vi "real time object finder single cam with save v1.0 EJA 09 14 2016.vi"() -> ()   [LabVIEW 2015]
doc: "The Low-Level Grab VI acquires images continuously and displays the images in an image control using low-level acquisition VIs. A grab is appropriate for high-speed applications in which you need to process only one image at a time."
uses:
  <vilib>/userdefined/High Color/IMAQdx.ctl
  <vilib>/vision/driver/IMAQdx.llb/IMAQdx Buffer Number Mode.ctl
  <vilib>/Utility/file.llb/Write To Spreadsheet File (DBL).vi
  <vilib>/vision/driver/NI_Vision_Acquisition_Software.lvlib
  <resource>/objmgr/imaqdx.rc
  <vilib>/Analysis/NI_AALBase.lvlib
panel:
  out "y position histogram":T1(graph)={"X Values"=[496.25, 512.75, 529.25, 545.75, 562.25, 578.75, 595.25, 611.75, 628.25, 644.75], "Histogram: h(x)"=[12, 8, 7, 11, 11, 133, 43, 197, 42, 41]}
  out "x position histogram":T1(graph)={"X Values"=[593.75, 617.25, 640.75, 664.25, 687.75, 711.25, 734.75, 758.25, 781.75, 805.25], "Histogram: h(x)"=[96, 9, 49, 4, 6, 45, 112, 75, 70, 39]}
  in  "histogram \nbins":i32=10
  in  "always save\non stop\nimaging":bool=TRUE
  in  "acquisition \ntime (s)":i32=5
  in  "save for a \ndesignated \nperiod":bool
  out "trajectory":cluster{i32[], i32[]}(graph)={[740, 740, 740, 740, 740, 740, 740, 740, 740, 740, 740, 740, 740, 740, 740, 740, 740, 740, 740, 740, 740, 740, 740, 740, 740, 740, 740, 740, 740, 740, 740, 740, 740, 740, 740, 740, 740, 740, 740, 740, 740, 740, 740, 740, 740, 740, 740, 740, 740, 741, 742, 744, 747, 749, 751, 752, 753, 755, 757, 759, 760, 763, 766, 771, 776, 779, 783, 787, 789, 790, 791, 791, 791, 790, 788, 785, 782, 778, 775, 773, 771, 770, 769, 767, 765, 763, 760, 755, 749, 744, 740, 736, 733, 730, 727, 725, 724, 723, 722, 722, 723, 726, 730, 733, 738, 743, 748, 752, 756, 758, 761, 764, 768, 770, 772, 776, 780, 783, 786, 788, 790, 790, 790, 789, 788, 786, 784, 781, 779, 776, 773, 769, 765, 760, 753, 746, 740, 735, 730, 725, 723, 721, 717, 713, 710, 707, 705, 703, 701, 700, 701, 701, 703, 705, 707, 710, 713, 718, 723, 728, 733, 738, 743, 750, 758, 762, 763, 765, 767, 769, 771, 773, 773, 773, 771, 769, 766, 763, 759, 756, 752, 749, 746, 743, 739, 736, 732, 727, 725, 724, 721, 719, 716, 714, 713, 712, 711, 710, 709, 709, 710, 710, 712, 715, 718, 721, 724, 728, 733, 740, 748, 755, 759, 763, 769, 773, 776, 779, 780, 780, 781, 780, 779, 778, 777, 775, 774, 772, 769, 769, 768, 766, 764, 762, 758, 755, 753, 748, 744, 741, 739, 734, 730, 727, 725, 723, 722, 722, 722, 722, 723, 724, 727, 729, 731, 734, 737, 741, 746, 750, 754, 757, 762, 764, 765, 765, 765, 765, 765, 767, 771, 776, 777, 780, 783, 785, 787, 790, 792, 794, 797, 798, 801, 804, 806, 808, 810, 811, 812, 814, 816, 817, 817, 817, 817, 817, 817, 817, 817, 817, 817, 817, 817, 817, 817, 817, 817, 817, 817, 817, 817, 817, 815, 813, 808, 804, 799, 794, 791, 789, 785, 782, 777, 772, 768, 765, 762, 759, 754, 747, 743, 739, 734, 728, 723, 719, 715, 711, 708, 705, 701, 697, 693, 689, 684, 681, 677, 673, 667, 658, 654, 652, 650, 647, 642, 640, 640, 638, 637, 637, 637, 637, 637, 637, 637, 636, 636, 636, 635, 635, 635, 635, 635, 634, 634, 633, 633, 633, 633, 633, 633, 633, 633, 634, 634, 635, 635, 636, 636, 637, 637, 638, 638, 639, 639, 639, 638, 634, 631, 629, 626, 623, 619, 616, 614, 612, 610, 608, 607, 605, 602, 600, 599, 597, 594, 592, 591, 589, 588, 587, 586, 585, 584, 583, 582, 582, 582, 582, 582, 582, 582, 584, 585, 585, 585, 585, 585, 585, 585, 585, 585, 585, 585, 585, 585, 585, 585, 585, 585, 585, 585, 585, 585, 585, 585, 585, 585, 585, 585, 585, 585, 585, 585, 585, 585, 585, 585, 585, 585, 585, 585, 585, 585, 585, 585, 585, 585, 585, 585, 585, 585, 585, 585, 585, 585, 585, 585, 585, 585, 585, 585, 585, 585, 585, 585, 585, 585, 585, 585, 585, 585, 585, 585, 585, 585], [615, 618, 617, 617, 617, 618, 617, 617, 617, 618, 618, 617, 617, 618, 618, 617, 618, 617, 618, 617, 619, 617, 618, 615, 617, 618, 618, 617, 619, 618, 618, 618, 618, 619, 617, 615, 617, 617, 615, 617, 618, 617, 617, 615, 615, 617, 617, 619, 618, 615, 614, 613, 613, 610, 610, 609, 608, 607, 607, 609, 608, 612, 612, 615, 616, 620, 622, 625, 620, 628, 630, 631, 633, 636, 639, 643, 647, 651, 652, 653, 653, 653, 653, 652, 653, 653, 652, 651, 647, 646, 644, 642, 644, 637, 636, 633, 633, 630, 625, 625, 622, 619, 616, 611, 607, 605, 604, 603, 602, 604, 602, 603, 601, 602, 604, 607, 610, 613, 616, 619, 622, 625, 628, 631, 636, 638, 639, 638, 639, 639, 642, 643, 643, 643, 645, 643, 644, 644, 646, 645, 650, 643, 646, 644, 640, 639, 636, 631, 627, 625, 620, 617, 614, 610, 607, 599, 596, 593, 591, 589, 584, 583, 584, 584, 583, 585, 588, 587, 589, 593, 598, 601, 602, 607, 610, 616, 618, 620, 622, 623, 625, 624, 629, 624, 624, 628, 625, 627, 625, 625, 624, 622, 625, 616, 614, 616, 613, 611, 607, 604, 595, 592, 590, 588, 586, 584, 583, 579, 576, 575, 576, 577, 579, 577, 580, 583, 585, 590, 592, 596, 599, 602, 608, 608, 612, 611, 612, 615, 615, 615, 616, 616, 616, 614, 616, 615, 617, 615, 613, 609, 609, 607, 604, 602, 600, 597, 595, 593, 591, 590, 589, 585, 587, 584, 583, 584, 579, 578, 576, 575, 574, 576, 572, 572, 575, 573, 575, 575, 573, 573, 574, 578, 576, 577, 578, 578, 581, 581, 581, 582, 583, 583, 584, 585, 579, 586, 587, 586, 583, 583, 583, 583, 583, 583, 583, 583, 583, 583, 583, 583, 583, 583, 583, 583, 583, 583, 583, 583, 583, 583, 583, 587, 583, 582, 586, 585, 585, 584, 584, 583, 583, 583, 582, 581, 583, 583, 580, 581, 581, 581, 579, 579, 578, 577, 576, 576, 580, 579, 579, 576, 577, 577, 577, 576, 576, 580, 575, 574, 578, 577, 575, 575, 575, 575, 576, 575, 575, 576, 575, 575, 575, 575, 574, 573, 570, 568, 564, 562, 560, 558, 555, 553, 549, 547, 545, 543, 541, 540, 538, 535, 530, 525, 525, 517, 517, 515, 507, 509, 503, 497, 499, 492, 490, 488, 488, 488, 489, 495, 498, 503, 509, 514, 519, 525, 530, 535, 541, 545, 550, 554, 558, 562, 567, 571, 576, 580, 583, 587, 593, 595, 598, 602, 605, 608, 611, 612, 612, 612, 612, 611, 612, 610, 609, 609, 609, 609, 609, 609, 609, 609, 609, 609, 609, 609, 609, 609, 609, 609, 609, 608, 609, 609, 609, 610, 609, 609, 609, 609, 609, 609, 609, 610, 609, 610, 609, 609, 613, 609, 613, 609, 609, 609, 611, 609, 609, 609, 609, 609, 608, 609, 609, 609, 609, 609, 609, 609, 609, 609, 609, 609, 609, 609, 609, 609, 609, 609, 609, 609, 609, 611, 609, 609, 609, 609, 608]}
  in  "save\nlast\nimage":bool
  in  "stop no save":bool
  out "date stub assigned":string="_2018Y_03M_05D_11h_28m_40s"
  in  "Acquire\ndata":bool
  in  "Experimental stub":string="test01_test"
  out "Saving":bool
  in  "save data":bool
  in  "save path":path=path "C:/Users/StangebyeTO1/OneDrive/Documents/RasterImageLabview/object_tracker"
  in  "number\nformat (%.6f)":string="%.6f"
  in  "Marker\nText color":u32(colorbox)=16711680
  out "Multiplot":cluster{cluster{dbl, i32}[]}[](graph)=[{[{0.0, 740}, {0.025, 740}, {0.049, 740}, {0.073, 740}, {0.097, 740}, {0.122, 740}, {0.145, 740}, {0.171, 740}, {0.194, 740}, {0.218, 740}, {0.242, 740}, {0.266, 740}, {0.29, 740}, {0.313, 740}, {0.338, 740}, {0.361, 740}, {0.385, 740}, {0.41, 740}, {0.434, 740}, {0.458, 740}, {0.483, 740}, {0.506, 740}, {0.53, 740}, {0.556, 740}, {0.578, 740}, {0.602, 740}, {0.626, 740}, {0.651, 740}, {0.674, 740}, {0.698, 740}, {0.722, 740}, {0.746, 740}, {0.771, 740}, {0.794, 740}, {0.819, 740}, {0.842, 740}, {0.867, 740}, {0.89, 740}, {0.915, 740}, {0.939, 740}, {0.963, 740}, {0.987, 740}, {1.011, 740}, {1.035, 740}, {1.059, 740}, {1.083, 740}, {1.107, 740}, {1.132, 740}, {1.157, 740}, {1.179, 741}, {1.204, 742}, {1.227, 744}, {1.251, 747}, {1.275, 749}, {1.3, 751}, {1.323, 752}, {1.348, 753}, {1.372, 755}, {1.396, 757}, {1.42, 759}, {1.444, 760}, {1.468, 763}, {1.492, 766}, {1.516, 771}, {1.54, 776}, {1.564, 779}, {1.588, 783}, {1.612, 787}, {1.637, 789}, {1.66, 790}, {1.685, 791}, {1.708, 791}, {1.733, 791}, {1.756, 790}, {1.78, 788}, {1.805, 785}, {1.828, 782}, {1.853, 778}, {1.876, 775}, {1.901, 773}, {1.925, 771}, {1.95, 770}, {1.973, 769}, {1.997, 767}, {2.021, 765}, {2.045, 763}, {2.07, 760}, {2.093, 755}, {2.118, 749}, {2.141, 744}, {2.166, 740}, {2.189, 736}, {2.213, 733}, {2.237, 730}, {2.261, 727}, {2.286, 725}, {2.31, 724}, {2.334, 723}, {2.357, 722}, {2.382, 722}, {2.406, 723}, {2.429, 726}, {2.454, 730}, {2.478, 733}, {2.503, 738}, {2.526, 743}, {2.55, 748}, {2.574, 752}, {2.598, 756}, {2.622, 758}, {2.646, 761}, {2.671, 764}, {2.694, 768}, {2.718, 770}, {2.743, 772}, {2.767, 776}, {2.791, 780}, {2.814, 783}, {2.838, 786}, {2.863, 788}, {2.886, 790}, {2.91, 790}, {2.935, 790}, {2.959, 789}, {2.984, 788}, {3.007, 786}, {3.031, 784}, {3.055, 781}, {3.079, 779}, {3.104, 776}, {3.127, 773}, {3.152, 769}, {3.175, 765}, {3.2, 760}, {3.225, 753}, {3.249, 746}, {3.272, 740}, {3.295, 735}, {3.32, 730}, {3.343, 725}, {3.368, 723}, {3.391, 721}, {3.415, 717}, {3.44, 713}, {3.463, 710}, {3.487, 707}, {3.512, 705}, {3.536, 703}, {3.56, 701}, {3.584, 700}, {3.608, 701}, {3.632, 701}, {3.657, 703}, {3.68, 705}, {3.704, 707}, {3.728, 710}, {3.753, 713}, {3.776, 718}, {3.801, 723}, {3.824, 728}, {3.849, 733}, {3.872, 738}, {3.897, 743}, {3.921, 750}, {3.944, 758}, {3.969, 762}, {3.993, 763}, {4.017, 765}, {4.04, 767}, {4.064, 769}, {4.089, 771}, {4.113, 773}, {4.138, 773}, {4.162, 773}, {4.186, 771}, {4.209, 769}, {4.234, 766}, {4.257, 763}, {4.281, 759}, {4.306, 756}, {4.33, 752}, {4.354, 749}, {4.377, 746}, {4.401, 743}, {4.426, 739}, {4.45, 736}, {4.474, 732}, {4.498, 727}, {4.522, 725}, {4.546, 724}, {4.57, 721}, {4.594, 719}, {4.618, 716}, {4.641, 714}, {4.668, 713}, {4.69, 712}, {4.714, 711}, {4.738, 710}, {4.762, 709}, {4.787, 709}, {4.81, 710}, {4.834, 710}, {4.86, 712}, {4.883, 715}, {4.906, 718}, {4.93, 721}, {4.955, 724}, {4.979, 728}, {5.003, 733}, {5.027, 740}, {5.051, 748}, {5.075, 755}, {5.099, 759}, {5.123, 763}, {5.147, 769}, {5.172, 773}, {5.195, 776}, {5.22, 779}, {5.245, 780}, {5.268, 780}, {5.291, 781}, {5.315, 780}, {5.339, 779}, {5.363, 778}, {5.388, 777}, {5.411, 775}, {5.436, 774}, {5.46, 772}, {5.484, 769}, {5.508, 769}, {5.531, 768}, {5.555, 766}, {5.58, 764}, {5.604, 762}, {5.628, 758}, {5.652, 755}, {5.676, 753}, {5.7, 748}, {5.724, 744}, {5.748, 741}, {5.772, 739}, {5.796, 734}, {5.821, 730}, {5.844, 727}, {5.868, 725}, {5.892, 723}, {5.917, 722}, {5.94, 722}, {5.966, 722}, {5.989, 722}, {6.013, 723}, {6.037, 724}, {6.06, 727}, {6.085, 729}, {6.108, 731}, {6.133, 734}, {6.158, 737}, {6.181, 741}, {6.205, 746}, {6.229, 750}, {6.254, 754}, {6.277, 757}, {6.301, 762}, {6.325, 764}, {6.35, 765}, {6.373, 765}, {6.397, 765}, {6.423, 765}, {6.446, 765}, {6.471, 767}, {6.494, 771}, {6.518, 776}, {6.542, 777}, {6.567, 780}, {6.59, 783}, {6.614, 785}, {6.638, 787}, {6.662, 790}, {6.687, 792}, {6.71, 794}, {6.734, 797}, {6.758, 798}, {6.783, 801}, {6.806, 804}, {6.83, 806}, {6.854, 808}, {6.878, 810}, {6.903, 811}, {6.926, 812}, {6.951, 814}, {6.974, 816}, {6.999, 817}, {7.023, 817}, {7.048, 817}, {7.071, 817}, {7.094, 817}, {7.12, 817}, {7.143, 817}, {7.168, 817}, {7.191, 817}, {7.215, 817}, {7.239, 817}, {7.263, 817}, {7.287, 817}, {7.311, 817}, {7.336, 817}, {7.359, 817}, {7.384, 817}, {7.407, 817}, {7.432, 817}, {7.456, 817}, {7.479, 817}, {7.504, 815}, {7.528, 813}, {7.552, 808}, {7.576, 804}, {7.6, 799}, {7.624, 794}, {7.648, 791}, {7.672, 789}, {7.696, 785}, {7.721, 782}, {7.744, 777}, {7.769, 772}, {7.792, 768}, {7.817, 765}, {7.84, 762}, {7.864, 759}, {7.888, 754}, {7.912, 747}, {7.936, 743}, {7.96, 739}, {7.984, 734}, {8.009, 728}, {8.033, 723}, {8.056, 719}, {8.081, 715}, {8.105, 711}, {8.128, 708}, {8.153, 705}, {8.176, 701}, {8.201, 697}, {8.224, 693}, {8.249, 689}, {8.273, 684}, {8.297, 681}, {8.321, 677}, {8.345, 673}, {8.369, 667}, {8.393, 658}, {8.417, 654}, {8.441, 652}, {8.465, 650}, {8.489, 647}, {8.513, 642}, {8.537, 640}, {8.561, 640}, {8.585, 638}, {8.609, 637}, {8.634, 637}, {8.657, 637}, {8.681, 637}, {8.706, 637}, {8.73, 637}, {8.754, 637}, {8.778, 636}, {8.802, 636}, {8.826, 636}, {8.851, 635}, {8.874, 635}, {8.899, 635}, {8.922, 635}, {8.947, 635}, {8.971, 634}, {8.995, 634}, {9.02, 633}, {9.042, 633}, {9.066, 633}, {9.09, 633}, {9.114, 633}, {9.139, 633}, {9.162, 633}, {9.188, 633}, {9.211, 634}, {9.236, 634}, {9.259, 635}, {9.283, 635}, {9.307, 636}, {9.332, 636}, {9.355, 637}, {9.379, 637}, {9.404, 638}, {9.427, 638}, {9.451, 639}, {9.475, 639}, {9.5, 639}, {9.523, 638}, {9.547, 634}, {9.572, 631}, {9.595, 629}, {9.62, 626}, {9.643, 623}, {9.668, 619}, {9.691, 616}, {9.715, 614}, {9.739, 612}, {9.764, 610}, {9.788, 608}, {9.812, 607}, {9.837, 605}, {9.86, 602}, {9.884, 600}, {9.908, 599}, {9.932, 597}, {9.955, 594}, {9.98, 592}, {10.004, 591}, {10.028, 589}, {10.053, 588}, {10.076, 587}, {10.101, 586}, {10.124, 585}, {10.149, 584}, {10.172, 583}, {10.196, 582}, {10.221, 582}, {10.244, 582}, {10.269, 582}, {10.293, 582}, {10.317, 582}, {10.341, 582}, {10.365, 584}, {10.39, 585}, {10.412, 585}, {10.437, 585}, {10.461, 585}, {10.485, 585}, {10.509, 585}, {10.534, 585}, {10.557, 585}, {10.581, 585}, {10.605, 585}, {10.629, 585}, {10.654, 585}, {10.677, 585}, {10.701, 585}, {10.725, 585}, {10.75, 585}, {10.773, 585}, {10.797, 585}, {10.822, 585}, {10.845, 585}, {10.87, 585}, {10.893, 585}, {10.918, 585}, {10.942, 585}, {10.966, 585}, {10.99, 585}, {11.014, 585}, {11.038, 585}, {11.062, 585}, {11.088, 585}, {11.11, 585}, {11.135, 585}, {11.159, 585}, {11.182, 585}, {11.207, 585}, {11.231, 585}, {11.255, 585}, {11.279, 585}, {11.303, 585}, {11.326, 585}, {11.353, 585}, {11.375, 585}, {11.4, 585}, {11.423, 585}, {11.448, 585}, {11.471, 585}, {11.495, 585}, {11.52, 585}, {11.543, 585}, {11.569, 585}, {11.602, 585}, {11.621, 585}, {11.641, 585}, {11.664, 585}, {11.688, 585}, {11.711, 585}, {11.736, 585}, {11.76, 585}, {11.784, 585}, {11.808, 585}, {11.831, 585}, {11.856, 585}, {11.879, 585}, {11.904, 585}, {11.928, 585}, {11.952, 585}, {11.975, 585}, {12.0, 585}, {12.024, 585}, {12.047, 585}, {12.072, 585}, {12.096, 585}, {12.121, 585}]}, {[{0.0, 615}, {0.025, 618}, {0.049, 617}, {0.073, 617}, {0.097, 617}, {0.122, 618}, {0.145, 617}, {0.171, 617}, {0.194, 617}, {0.218, 618}, {0.242, 618}, {0.266, 617}, {0.29, 617}, {0.313, 618}, {0.338, 618}, {0.361, 617}, {0.385, 618}, {0.41, 617}, {0.434, 618}, {0.458, 617}, {0.483, 619}, {0.506, 617}, {0.53, 618}, {0.556, 615}, {0.578, 617}, {0.602, 618}, {0.626, 618}, {0.651, 617}, {0.674, 619}, {0.698, 618}, {0.722, 618}, {0.746, 618}, {0.771, 618}, {0.794, 619}, {0.819, 617}, {0.842, 615}, {0.867, 617}, {0.89, 617}, {0.915, 615}, {0.939, 617}, {0.963, 618}, {0.987, 617}, {1.011, 617}, {1.035, 615}, {1.059, 615}, {1.083, 617}, {1.107, 617}, {1.132, 619}, {1.157, 618}, {1.179, 615}, {1.204, 614}, {1.227, 613}, {1.251, 613}, {1.275, 610}, {1.3, 610}, {1.323, 609}, {1.348, 608}, {1.372, 607}, {1.396, 607}, {1.42, 609}, {1.444, 608}, {1.468, 612}, {1.492, 612}, {1.516, 615}, {1.54, 616}, {1.564, 620}, {1.588, 622}, {1.612, 625}, {1.637, 620}, {1.66, 628}, {1.685, 630}, {1.708, 631}, {1.733, 633}, {1.756, 636}, {1.78, 639}, {1.805, 643}, {1.828, 647}, {1.853, 651}, {1.876, 652}, {1.901, 653}, {1.925, 653}, {1.95, 653}, {1.973, 653}, {1.997, 652}, {2.021, 653}, {2.045, 653}, {2.07, 652}, {2.093, 651}, {2.118, 647}, {2.141, 646}, {2.166, 644}, {2.189, 642}, {2.213, 644}, {2.237, 637}, {2.261, 636}, {2.286, 633}, {2.31, 633}, {2.334, 630}, {2.357, 625}, {2.382, 625}, {2.406, 622}, {2.429, 619}, {2.454, 616}, {2.478, 611}, {2.503, 607}, {2.526, 605}, {2.55, 604}, {2.574, 603}, {2.598, 602}, {2.622, 604}, {2.646, 602}, {2.671, 603}, {2.694, 601}, {2.718, 602}, {2.743, 604}, {2.767, 607}, {2.791, 610}, {2.814, 613}, {2.838, 616}, {2.863, 619}, {2.886, 622}, {2.91, 625}, {2.935, 628}, {2.959, 631}, {2.984, 636}, {3.007, 638}, {3.031, 639}, {3.055, 638}, {3.079, 639}, {3.104, 639}, {3.127, 642}, {3.152, 643}, {3.175, 643}, {3.2, 643}, {3.225, 645}, {3.249, 643}, {3.272, 644}, {3.295, 644}, {3.32, 646}, {3.343, 645}, {3.368, 650}, {3.391, 643}, {3.415, 646}, {3.44, 644}, {3.463, 640}, {3.487, 639}, {3.512, 636}, {3.536, 631}, {3.56, 627}, {3.584, 625}, {3.608, 620}, {3.632, 617}, {3.657, 614}, {3.68, 610}, {3.704, 607}, {3.728, 599}, {3.753, 596}, {3.776, 593}, {3.801, 591}, {3.824, 589}, {3.849, 584}, {3.872, 583}, {3.897, 584}, {3.921, 584}, {3.944, 583}, {3.969, 585}, {3.993, 588}, {4.017, 587}, {4.04, 589}, {4.064, 593}, {4.089, 598}, {4.113, 601}, {4.138, 602}, {4.162, 607}, {4.186, 610}, {4.209, 616}, {4.234, 618}, {4.257, 620}, {4.281, 622}, {4.306, 623}, {4.33, 625}, {4.354, 624}, {4.377, 629}, {4.401, 624}, {4.426, 624}, {4.45, 628}, {4.474, 625}, {4.498, 627}, {4.522, 625}, {4.546, 625}, {4.57, 624}, {4.594, 622}, {4.618, 625}, {4.641, 616}, {4.668, 614}, {4.69, 616}, {4.714, 613}, {4.738, 611}, {4.762, 607}, {4.787, 604}, {4.81, 595}, {4.834, 592}, {4.86, 590}, {4.883, 588}, {4.906, 586}, {4.93, 584}, {4.955, 583}, {4.979, 579}, {5.003, 576}, {5.027, 575}, {5.051, 576}, {5.075, 577}, {5.099, 579}, {5.123, 577}, {5.147, 580}, {5.172, 583}, {5.195, 585}, {5.22, 590}, {5.245, 592}, {5.268, 596}, {5.291, 599}, {5.315, 602}, {5.339, 608}, {5.363, 608}, {5.388, 612}, {5.411, 611}, {5.436, 612}, {5.46, 615}, {5.484, 615}, {5.508, 615}, {5.531, 616}, {5.555, 616}, {5.58, 616}, {5.604, 614}, {5.628, 616}, {5.652, 615}, {5.676, 617}, {5.7, 615}, {5.724, 613}, {5.748, 609}, {5.772, 609}, {5.796, 607}, {5.821, 604}, {5.844, 602}, {5.868, 600}, {5.892, 597}, {5.917, 595}, {5.94, 593}, {5.966, 591}, {5.989, 590}, {6.013, 589}, {6.037, 585}, {6.06, 587}, {6.085, 584}, {6.108, 583}, {6.133, 584}, {6.158, 579}, {6.181, 578}, {6.205, 576}, {6.229, 575}, {6.254, 574}, {6.277, 576}, {6.301, 572}, {6.325, 572}, {6.35, 575}, {6.373, 573}, {6.397, 575}, {6.423, 575}, {6.446, 573}, {6.471, 573}, {6.494, 574}, {6.518, 578}, {6.542, 576}, {6.567, 577}, {6.59, 578}, {6.614, 578}, {6.638, 581}, {6.662, 581}, {6.687, 581}, {6.71, 582}, {6.734, 583}, {6.758, 583}, {6.783, 584}, {6.806, 585}, {6.83, 579}, {6.854, 586}, {6.878, 587}, {6.903, 586}, {6.926, 583}, {6.951, 583}, {6.974, 583}, {6.999, 583}, {7.023, 583}, {7.048, 583}, {7.071, 583}, {7.094, 583}, {7.12, 583}, {7.143, 583}, {7.168, 583}, {7.191, 583}, {7.215, 583}, {7.239, 583}, {7.263, 583}, {7.287, 583}, {7.311, 583}, {7.336, 583}, {7.359, 583}, {7.384, 583}, {7.407, 583}, {7.432, 583}, {7.456, 583}, {7.479, 587}, {7.504, 583}, {7.528, 582}, {7.552, 586}, {7.576, 585}, {7.6, 585}, {7.624, 584}, {7.648, 584}, {7.672, 583}, {7.696, 583}, {7.721, 583}, {7.744, 582}, {7.769, 581}, {7.792, 583}, {7.817, 583}, {7.84, 580}, {7.864, 581}, {7.888, 581}, {7.912, 581}, {7.936, 579}, {7.96, 579}, {7.984, 578}, {8.009, 577}, {8.033, 576}, {8.056, 576}, {8.081, 580}, {8.105, 579}, {8.128, 579}, {8.153, 576}, {8.176, 577}, {8.201, 577}, {8.224, 577}, {8.249, 576}, {8.273, 576}, {8.297, 580}, {8.321, 575}, {8.345, 574}, {8.369, 578}, {8.393, 577}, {8.417, 575}, {8.441, 575}, {8.465, 575}, {8.489, 575}, {8.513, 576}, {8.537, 575}, {8.561, 575}, {8.585, 576}, {8.609, 575}, {8.634, 575}, {8.657, 575}, {8.681, 575}, {8.706, 574}, {8.73, 573}, {8.754, 570}, {8.778, 568}, {8.802, 564}, {8.826, 562}, {8.851, 560}, {8.874, 558}, {8.899, 555}, {8.922, 553}, {8.947, 549}, {8.971, 547}, {8.995, 545}, {9.02, 543}, {9.042, 541}, {9.066, 540}, {9.09, 538}, {9.114, 535}, {9.139, 530}, {9.162, 525}, {9.188, 525}, {9.211, 517}, {9.236, 517}, {9.259, 515}, {9.283, 507}, {9.307, 509}, {9.332, 503}, {9.355, 497}, {9.379, 499}, {9.404, 492}, {9.427, 490}, {9.451, 488}, {9.475, 488}, {9.5, 488}, {9.523, 489}, {9.547, 495}, {9.572, 498}, {9.595, 503}, {9.62, 509}, {9.643, 514}, {9.668, 519}, {9.691, 525}, {9.715, 530}, {9.739, 535}, {9.764, 541}, {9.788, 545}, {9.812, 550}, {9.837, 554}, {9.86, 558}, {9.884, 562}, {9.908, 567}, {9.932, 571}, {9.955, 576}, {9.98, 580}, {10.004, 583}, {10.028, 587}, {10.053, 593}, {10.076, 595}, {10.101, 598}, {10.124, 602}, {10.149, 605}, {10.172, 608}, {10.196, 611}, {10.221, 612}, {10.244, 612}, {10.269, 612}, {10.293, 612}, {10.317, 611}, {10.341, 612}, {10.365, 610}, {10.39, 609}, {10.412, 609}, {10.437, 609}, {10.461, 609}, {10.485, 609}, {10.509, 609}, {10.534, 609}, {10.557, 609}, {10.581, 609}, {10.605, 609}, {10.629, 609}, {10.654, 609}, {10.677, 609}, {10.701, 609}, {10.725, 609}, {10.75, 609}, {10.773, 609}, {10.797, 608}, {10.822, 609}, {10.845, 609}, {10.87, 609}, {10.893, 610}, {10.918, 609}, {10.942, 609}, {10.966, 609}, {10.99, 609}, {11.014, 609}, {11.038, 609}, {11.062, 609}, {11.088, 610}, {11.11, 609}, {11.135, 610}, {11.159, 609}, {11.182, 609}, {11.207, 613}, {11.231, 609}, {11.255, 613}, {11.279, 609}, {11.303, 609}, {11.326, 609}, {11.353, 611}, {11.375, 609}, {11.4, 609}, {11.423, 609}, {11.448, 609}, {11.471, 609}, {11.495, 608}, {11.52, 609}, {11.543, 609}, {11.569, 609}, {11.602, 609}, {11.621, 609}, {11.641, 609}, {11.664, 609}, {11.688, 609}, {11.711, 609}, {11.736, 609}, {11.76, 609}, {11.784, 609}, {11.808, 609}, {11.831, 609}, {11.856, 609}, {11.879, 609}, {11.904, 609}, {11.928, 609}, {11.952, 609}, {11.975, 609}, {12.0, 611}, {12.024, 609}, {12.047, 609}, {12.072, 609}, {12.096, 609}, {12.121, 608}]}]
  out "FPS":i32=42
  out "time (s)":dbl[](array[numeric])=[0.0, 0.025, 0.049, 0.073, 0.097, 0.122, 0.145, 0.171, 0.194, 0.218, 0.242, 0.266, 0.29, 0.313, 0.338, 0.361, 0.385, 0.41, 0.434, 0.458, 0.483, 0.506, 0.53, 0.556, 0.578, 0.602, 0.626, 0.651, 0.674, 0.698, 0.722, 0.746, 0.771, 0.794, 0.819, 0.842, 0.867, 0.89, 0.915, 0.939, 0.963, 0.987, 1.011, 1.035, 1.059, 1.083, 1.107, 1.132, 1.157, 1.179, 1.204, 1.227, 1.251, 1.275, 1.3, 1.323, 1.348, 1.372, 1.396, 1.42, 1.444, 1.468, 1.492, 1.516, 1.54, 1.564, 1.588, 1.612, 1.637, 1.66, 1.685, 1.708, 1.733, 1.756, 1.78, 1.805, 1.828, 1.853, 1.876, 1.901, 1.925, 1.95, 1.973, 1.997, 2.021, 2.045, 2.07, 2.093, 2.118, 2.141, 2.166, 2.189, 2.213, 2.237, 2.261, 2.286, 2.31, 2.334, 2.357, 2.382, 2.406, 2.429, 2.454, 2.478, 2.503, 2.526, 2.55, 2.574, 2.598, 2.622, 2.646, 2.671, 2.694, 2.718, 2.743, 2.767, 2.791, 2.814, 2.838, 2.863, 2.886, 2.91, 2.935, 2.959, 2.984, 3.007, 3.031, 3.055, 3.079, 3.104, 3.127, 3.152, 3.175, 3.2, 3.225, 3.249, 3.272, 3.295, 3.32, 3.343, 3.368, 3.391, 3.415, 3.44, 3.463, 3.487, 3.512, 3.536, 3.56, 3.584, 3.608, 3.632, 3.657, 3.68, 3.704, 3.728, 3.753, 3.776, 3.801, 3.824, 3.849, 3.872, 3.897, 3.921, 3.944, 3.969, 3.993, 4.017, 4.04, 4.064, 4.089, 4.113, 4.138, 4.162, 4.186, 4.209, 4.234, 4.257, 4.281, 4.306, 4.33, 4.354, 4.377, 4.401, 4.426, 4.45, 4.474, 4.498, 4.522, 4.546, 4.57, 4.594, 4.618, 4.641, 4.668, 4.69, 4.714, 4.738, 4.762, 4.787, 4.81, 4.834, 4.86, 4.883, 4.906, 4.93, 4.955, 4.979, 5.003, 5.027, 5.051, 5.075, 5.099, 5.123, 5.147, 5.172, 5.195, 5.22, 5.245, 5.268, 5.291, 5.315, 5.339, 5.363, 5.388, 5.411, 5.436, 5.46, 5.484, 5.508, 5.531, 5.555, 5.58, 5.604, 5.628, 5.652, 5.676, 5.7, 5.724, 5.748, 5.772, 5.796, 5.821, 5.844, 5.868, 5.892, 5.917, 5.94, 5.966, 5.989, 6.013, 6.037, 6.06, 6.085, 6.108, 6.133, 6.158, 6.181, 6.205, 6.229, 6.254, 6.277, 6.301, 6.325, 6.35, 6.373, 6.397, 6.423, 6.446, 6.471, 6.494, 6.518, 6.542, 6.567, 6.59, 6.614, 6.638, 6.662, 6.687, 6.71, 6.734, 6.758, 6.783, 6.806, 6.83, 6.854, 6.878, 6.903, 6.926, 6.951, 6.974, 6.999, 7.023, 7.048, 7.071, 7.094, 7.12, 7.143, 7.168, 7.191, 7.215, 7.239, 7.263, 7.287, 7.311, 7.336, 7.359, 7.384, 7.407, 7.432, 7.456, 7.479, 7.504, 7.528, 7.552, 7.576, 7.6, 7.624, 7.648, 7.672, 7.696, 7.721, 7.744, 7.769, 7.792, 7.817, 7.84, 7.864, 7.888, 7.912, 7.936, 7.96, 7.984, 8.009, 8.033, 8.056, 8.081, 8.105, 8.128, 8.153, 8.176, 8.201, 8.224, 8.249, 8.273, 8.297, 8.321, 8.345, 8.369, 8.393, 8.417, 8.441, 8.465, 8.489, 8.513, 8.537, 8.561, 8.585, 8.609, 8.634, 8.657, 8.681, 8.706, 8.73, 8.754, 8.778, 8.802, 8.826, 8.851, 8.874, 8.899, 8.922, 8.947, 8.971, 8.995, 9.02, 9.042, 9.066, 9.09, 9.114, 9.139, 9.162, 9.188, 9.211, 9.236, 9.259, 9.283, 9.307, 9.332, 9.355, 9.379, 9.404, 9.427, 9.451, 9.475, 9.5, 9.523, 9.547, 9.572, 9.595, 9.62, 9.643, 9.668, 9.691, 9.715, 9.739, 9.764, 9.788, 9.812, 9.837, 9.86, 9.884, 9.908, 9.932, 9.955, 9.98, 10.004, 10.028, 10.053, 10.076, 10.101, 10.124, 10.149, 10.172, 10.196, 10.221, 10.244, 10.269, 10.293, 10.317, 10.341, 10.365, 10.39, 10.412, 10.437, 10.461, 10.485, 10.509, 10.534, 10.557, 10.581, 10.605, 10.629, 10.654, 10.677, 10.701, 10.725, 10.75, 10.773, 10.797, 10.822, 10.845, 10.87, 10.893, 10.918, 10.942, 10.966, 10.99, 11.014, 11.038, 11.062, 11.088, 11.11, 11.135, 11.159, 11.182, 11.207, 11.231, 11.255, 11.279, 11.303, 11.326, 11.353, 11.375, 11.4, 11.423, 11.448, 11.471, 11.495, 11.52, 11.543, 11.569, 11.602, 11.621, 11.641, 11.664, 11.688, 11.711, 11.736, 11.76, 11.784, 11.808, 11.831, 11.856, 11.879, 11.904, 11.928, 11.952, 11.975, 12.0, 12.024, 12.047, 12.072, 12.096, 12.121] format="%.3f"
  in  "Origin":cluster{"X":i32, "Y":i32}
  out "Y position vs time":cluster{dbl[], i32[]}(graph)={array[505 elements], [615, 618, 617, 617, 617, 618, 617, 617, 617, 618, 618, 617, 617, 618, 618, 617, 618, 617, 618, 617, 619, 617, 618, 615, 617, 618, 618, 617, 619, 618, 618, 618, 618, 619, 617, 615, 617, 617, 615, 617, 618, 617, 617, 615, 615, 617, 617, 619, 618, 615, 614, 613, 613, 610, 610, 609, 608, 607, 607, 609, 608, 612, 612, 615, 616, 620, 622, 625, 620, 628, 630, 631, 633, 636, 639, 643, 647, 651, 652, 653, 653, 653, 653, 652, 653, 653, 652, 651, 647, 646, 644, 642, 644, 637, 636, 633, 633, 630, 625, 625, 622, 619, 616, 611, 607, 605, 604, 603, 602, 604, 602, 603, 601, 602, 604, 607, 610, 613, 616, 619, 622, 625, 628, 631, 636, 638, 639, 638, 639, 639, 642, 643, 643, 643, 645, 643, 644, 644, 646, 645, 650, 643, 646, 644, 640, 639, 636, 631, 627, 625, 620, 617, 614, 610, 607, 599, 596, 593, 591, 589, 584, 583, 584, 584, 583, 585, 588, 587, 589, 593, 598, 601, 602, 607, 610, 616, 618, 620, 622, 623, 625, 624, 629, 624, 624, 628, 625, 627, 625, 625, 624, 622, 625, 616, 614, 616, 613, 611, 607, 604, 595, 592, 590, 588, 586, 584, 583, 579, 576, 575, 576, 577, 579, 577, 580, 583, 585, 590, 592, 596, 599, 602, 608, 608, 612, 611, 612, 615, 615, 615, 616, 616, 616, 614, 616, 615, 617, 615, 613, 609, 609, 607, 604, 602, 600, 597, 595, 593, 591, 590, 589, 585, 587, 584, 583, 584, 579, 578, 576, 575, 574, 576, 572, 572, 575, 573, 575, 575, 573, 573, 574, 578, 576, 577, 578, 578, 581, 581, 581, 582, 583, 583, 584, 585, 579, 586, 587, 586, 583, 583, 583, 583, 583, 583, 583, 583, 583, 583, 583, 583, 583, 583, 583, 583, 583, 583, 583, 583, 583, 583, 583, 587, 583, 582, 586, 585, 585, 584, 584, 583, 583, 583, 582, 581, 583, 583, 580, 581, 581, 581, 579, 579, 578, 577, 576, 576, 580, 579, 579, 576, 577, 577, 577, 576, 576, 580, 575, 574, 578, 577, 575, 575, 575, 575, 576, 575, 575, 576, 575, 575, 575, 575, 574, 573, 570, 568, 564, 562, 560, 558, 555, 553, 549, 547, 545, 543, 541, 540, 538, 535, 530, 525, 525, 517, 517, 515, 507, 509, 503, 497, 499, 492, 490, 488, 488, 488, 489, 495, 498, 503, 509, 514, 519, 525, 530, 535, 541, 545, 550, 554, 558, 562, 567, 571, 576, 580, 583, 587, 593, 595, 598, 602, 605, 608, 611, 612, 612, 612, 612, 611, 612, 610, 609, 609, 609, 609, 609, 609, 609, 609, 609, 609, 609, 609, 609, 609, 609, 609, 609, 608, 609, 609, 609, 610, 609, 609, 609, 609, 609, 609, 609, 610, 609, 610, 609, 609, 613, 609, 613, 609, 609, 609, 611, 609, 609, 609, 609, 609, 608, 609, 609, 609, 609, 609, 609, 609, 609, 609, 609, 609, 609, 609, 609, 609, 609, 609, 609, 609, 609, 611, 609, 609, 609, 609, 608]}
  out "X position vs time":cluster{dbl[], i32[]}(graph)={array[505 elements], [740, 740, 740, 740, 740, 740, 740, 740, 740, 740, 740, 740, 740, 740, 740, 740, 740, 740, 740, 740, 740, 740, 740, 740, 740, 740, 740, 740, 740, 740, 740, 740, 740, 740, 740, 740, 740, 740, 740, 740, 740, 740, 740, 740, 740, 740, 740, 740, 740, 741, 742, 744, 747, 749, 751, 752, 753, 755, 757, 759, 760, 763, 766, 771, 776, 779, 783, 787, 789, 790, 791, 791, 791, 790, 788, 785, 782, 778, 775, 773, 771, 770, 769, 767, 765, 763, 760, 755, 749, 744, 740, 736, 733, 730, 727, 725, 724, 723, 722, 722, 723, 726, 730, 733, 738, 743, 748, 752, 756, 758, 761, 764, 768, 770, 772, 776, 780, 783, 786, 788, 790, 790, 790, 789, 788, 786, 784, 781, 779, 776, 773, 769, 765, 760, 753, 746, 740, 735, 730, 725, 723, 721, 717, 713, 710, 707, 705, 703, 701, 700, 701, 701, 703, 705, 707, 710, 713, 718, 723, 728, 733, 738, 743, 750, 758, 762, 763, 765, 767, 769, 771, 773, 773, 773, 771, 769, 766, 763, 759, 756, 752, 749, 746, 743, 739, 736, 732, 727, 725, 724, 721, 719, 716, 714, 713, 712, 711, 710, 709, 709, 710, 710, 712, 715, 718, 721, 724, 728, 733, 740, 748, 755, 759, 763, 769, 773, 776, 779, 780, 780, 781, 780, 779, 778, 777, 775, 774, 772, 769, 769, 768, 766, 764, 762, 758, 755, 753, 748, 744, 741, 739, 734, 730, 727, 725, 723, 722, 722, 722, 722, 723, 724, 727, 729, 731, 734, 737, 741, 746, 750, 754, 757, 762, 764, 765, 765, 765, 765, 765, 767, 771, 776, 777, 780, 783, 785, 787, 790, 792, 794, 797, 798, 801, 804, 806, 808, 810, 811, 812, 814, 816, 817, 817, 817, 817, 817, 817, 817, 817, 817, 817, 817, 817, 817, 817, 817, 817, 817, 817, 817, 817, 817, 815, 813, 808, 804, 799, 794, 791, 789, 785, 782, 777, 772, 768, 765, 762, 759, 754, 747, 743, 739, 734, 728, 723, 719, 715, 711, 708, 705, 701, 697, 693, 689, 684, 681, 677, 673, 667, 658, 654, 652, 650, 647, 642, 640, 640, 638, 637, 637, 637, 637, 637, 637, 637, 636, 636, 636, 635, 635, 635, 635, 635, 634, 634, 633, 633, 633, 633, 633, 633, 633, 633, 634, 634, 635, 635, 636, 636, 637, 637, 638, 638, 639, 639, 639, 638, 634, 631, 629, 626, 623, 619, 616, 614, 612, 610, 608, 607, 605, 602, 600, 599, 597, 594, 592, 591, 589, 588, 587, 586, 585, 584, 583, 582, 582, 582, 582, 582, 582, 582, 584, 585, 585, 585, 585, 585, 585, 585, 585, 585, 585, 585, 585, 585, 585, 585, 585, 585, 585, 585, 585, 585, 585, 585, 585, 585, 585, 585, 585, 585, 585, 585, 585, 585, 585, 585, 585, 585, 585, 585, 585, 585, 585, 585, 585, 585, 585, 585, 585, 585, 585, 585, 585, 585, 585, 585, 585, 585, 585, 585, 585, 585, 585, 585, 585, 585, 585, 585, 585, 585, 585, 585, 585, 585]}
  in  "Pixel intensity\nthreshold":i32=200
  in  "Row min":i32=100
  in  "Row max":i32=1150
  in  "Column min":i32=100
  in  "Column max":i32=1800
  out "X positions\ncamera 1\n(image \ncoordinates)":i32[](array[numeric])=[740, 740, 740, 740, 740, 740, 740, 740, 740, 740, 740, 740, 740, 740, 740, 740, 740, 740, 740, 740, 740, 740, 740, 740, 740, 740, 740, 740, 740, 740, 740, 740, 740, 740, 740, 740, 740, 740, 740, 740, 740, 740, 740, 740, 740, 740, 740, 740, 740, 741, 742, 744, 747, 749, 751, 752, 753, 755, 757, 759, 760, 763, 766, 771, 776, 779, 783, 787, 789, 790, 791, 791, 791, 790, 788, 785, 782, 778, 775, 773, 771, 770, 769, 767, 765, 763, 760, 755, 749, 744, 740, 736, 733, 730, 727, 725, 724, 723, 722, 722, 723, 726, 730, 733, 738, 743, 748, 752, 756, 758, 761, 764, 768, 770, 772, 776, 780, 783, 786, 788, 790, 790, 790, 789, 788, 786, 784, 781, 779, 776, 773, 769, 765, 760, 753, 746, 740, 735, 730, 725, 723, 721, 717, 713, 710, 707, 705, 703, 701, 700, 701, 701, 703, 705, 707, 710, 713, 718, 723, 728, 733, 738, 743, 750, 758, 762, 763, 765, 767, 769, 771, 773, 773, 773, 771, 769, 766, 763, 759, 756, 752, 749, 746, 743, 739, 736, 732, 727, 725, 724, 721, 719, 716, 714, 713, 712, 711, 710, 709, 709, 710, 710, 712, 715, 718, 721, 724, 728, 733, 740, 748, 755, 759, 763, 769, 773, 776, 779, 780, 780, 781, 780, 779, 778, 777, 775, 774, 772, 769, 769, 768, 766, 764, 762, 758, 755, 753, 748, 744, 741, 739, 734, 730, 727, 725, 723, 722, 722, 722, 722, 723, 724, 727, 729, 731, 734, 737, 741, 746, 750, 754, 757, 762, 764, 765, 765, 765, 765, 765, 767, 771, 776, 777, 780, 783, 785, 787, 790, 792, 794, 797, 798, 801, 804, 806, 808, 810, 811, 812, 814, 816, 817, 817, 817, 817, 817, 817, 817, 817, 817, 817, 817, 817, 817, 817, 817, 817, 817, 817, 817, 817, 817, 815, 813, 808, 804, 799, 794, 791, 789, 785, 782, 777, 772, 768, 765, 762, 759, 754, 747, 743, 739, 734, 728, 723, 719, 715, 711, 708, 705, 701, 697, 693, 689, 684, 681, 677, 673, 667, 658, 654, 652, 650, 647, 642, 640, 640, 638, 637, 637, 637, 637, 637, 637, 637, 636, 636, 636, 635, 635, 635, 635, 635, 634, 634, 633, 633, 633, 633, 633, 633, 633, 633, 634, 634, 635, 635, 636, 636, 637, 637, 638, 638, 639, 639, 639, 638, 634, 631, 629, 626, 623, 619, 616, 614, 612, 610, 608, 607, 605, 602, 600, 599, 597, 594, 592, 591, 589, 588, 587, 586, 585, 584, 583, 582, 582, 582, 582, 582, 582, 582, 584, 585, 585, 585, 585, 585, 585, 585, 585, 585, 585, 585, 585, 585, 585, 585, 585, 585, 585, 585, 585, 585, 585, 585, 585, 585, 585, 585, 585, 585, 585, 585, 585, 585, 585, 585, 585, 585, 585, 585, 585, 585, 585, 585, 585, 585, 585, 585, 585, 585, 585, 585, 585, 585, 585, 585, 585, 585, 585, 585, 585, 585, 585, 585, 585, 585, 585, 585, 585, 585, 585, 585, 585, 585]
  out "Y positions camera 1 \n(image \ncoordinates)":i32[](array[numeric])=[615, 618, 617, 617, 617, 618, 617, 617, 617, 618, 618, 617, 617, 618, 618, 617, 618, 617, 618, 617, 619, 617, 618, 615, 617, 618, 618, 617, 619, 618, 618, 618, 618, 619, 617, 615, 617, 617, 615, 617, 618, 617, 617, 615, 615, 617, 617, 619, 618, 615, 614, 613, 613, 610, 610, 609, 608, 607, 607, 609, 608, 612, 612, 615, 616, 620, 622, 625, 620, 628, 630, 631, 633, 636, 639, 643, 647, 651, 652, 653, 653, 653, 653, 652, 653, 653, 652, 651, 647, 646, 644, 642, 644, 637, 636, 633, 633, 630, 625, 625, 622, 619, 616, 611, 607, 605, 604, 603, 602, 604, 602, 603, 601, 602, 604, 607, 610, 613, 616, 619, 622, 625, 628, 631, 636, 638, 639, 638, 639, 639, 642, 643, 643, 643, 645, 643, 644, 644, 646, 645, 650, 643, 646, 644, 640, 639, 636, 631, 627, 625, 620, 617, 614, 610, 607, 599, 596, 593, 591, 589, 584, 583, 584, 584, 583, 585, 588, 587, 589, 593, 598, 601, 602, 607, 610, 616, 618, 620, 622, 623, 625, 624, 629, 624, 624, 628, 625, 627, 625, 625, 624, 622, 625, 616, 614, 616, 613, 611, 607, 604, 595, 592, 590, 588, 586, 584, 583, 579, 576, 575, 576, 577, 579, 577, 580, 583, 585, 590, 592, 596, 599, 602, 608, 608, 612, 611, 612, 615, 615, 615, 616, 616, 616, 614, 616, 615, 617, 615, 613, 609, 609, 607, 604, 602, 600, 597, 595, 593, 591, 590, 589, 585, 587, 584, 583, 584, 579, 578, 576, 575, 574, 576, 572, 572, 575, 573, 575, 575, 573, 573, 574, 578, 576, 577, 578, 578, 581, 581, 581, 582, 583, 583, 584, 585, 579, 586, 587, 586, 583, 583, 583, 583, 583, 583, 583, 583, 583, 583, 583, 583, 583, 583, 583, 583, 583, 583, 583, 583, 583, 583, 583, 587, 583, 582, 586, 585, 585, 584, 584, 583, 583, 583, 582, 581, 583, 583, 580, 581, 581, 581, 579, 579, 578, 577, 576, 576, 580, 579, 579, 576, 577, 577, 577, 576, 576, 580, 575, 574, 578, 577, 575, 575, 575, 575, 576, 575, 575, 576, 575, 575, 575, 575, 574, 573, 570, 568, 564, 562, 560, 558, 555, 553, 549, 547, 545, 543, 541, 540, 538, 535, 530, 525, 525, 517, 517, 515, 507, 509, 503, 497, 499, 492, 490, 488, 488, 488, 489, 495, 498, 503, 509, 514, 519, 525, 530, 535, 541, 545, 550, 554, 558, 562, 567, 571, 576, 580, 583, 587, 593, 595, 598, 602, 605, 608, 611, 612, 612, 612, 612, 611, 612, 610, 609, 609, 609, 609, 609, 609, 609, 609, 609, 609, 609, 609, 609, 609, 609, 609, 609, 608, 609, 609, 609, 610, 609, 609, 609, 609, 609, 609, 609, 610, 609, 610, 609, 609, 613, 609, 613, 609, 609, 609, 611, 609, 609, 609, 609, 609, 608, 609, 609, 609, 609, 609, 609, 609, 609, 609, 609, 609, 609, 609, 609, 609, 609, 609, 609, 609, 609, 611, 609, 609, 609, 609, 608]
  out "LIVE":bool
  in  "stop":bool
  out "Camera backlog":i32(slide)=-1 scale=0.0..50.0
  in  "IMAQdx Device Camera":T2="cam0"
  in  "Buffers Camera 1":u32=50
  out "Image":T3(plugin-control)
  # "PROGRAM INFO\n\nThis program finds the\nfirst pixel below the \nuser threshold in\nthe user specified\nROI below"
  # "Camera search ROI"
  # "Data acquisition \nsettings"
  # "issues\n\nHow do we know if frames \nare dropped?\n\nProbably will need to save data\nin sections to an open file\n\nCould have a sliding ROI based\non previous trailing edge position\n\nCould process each data chunk\nseparately to avoid frame dropping\nissues.  I.e. if you write every 1000\npoints, then in post processing only\nprocess 1000 at a time."
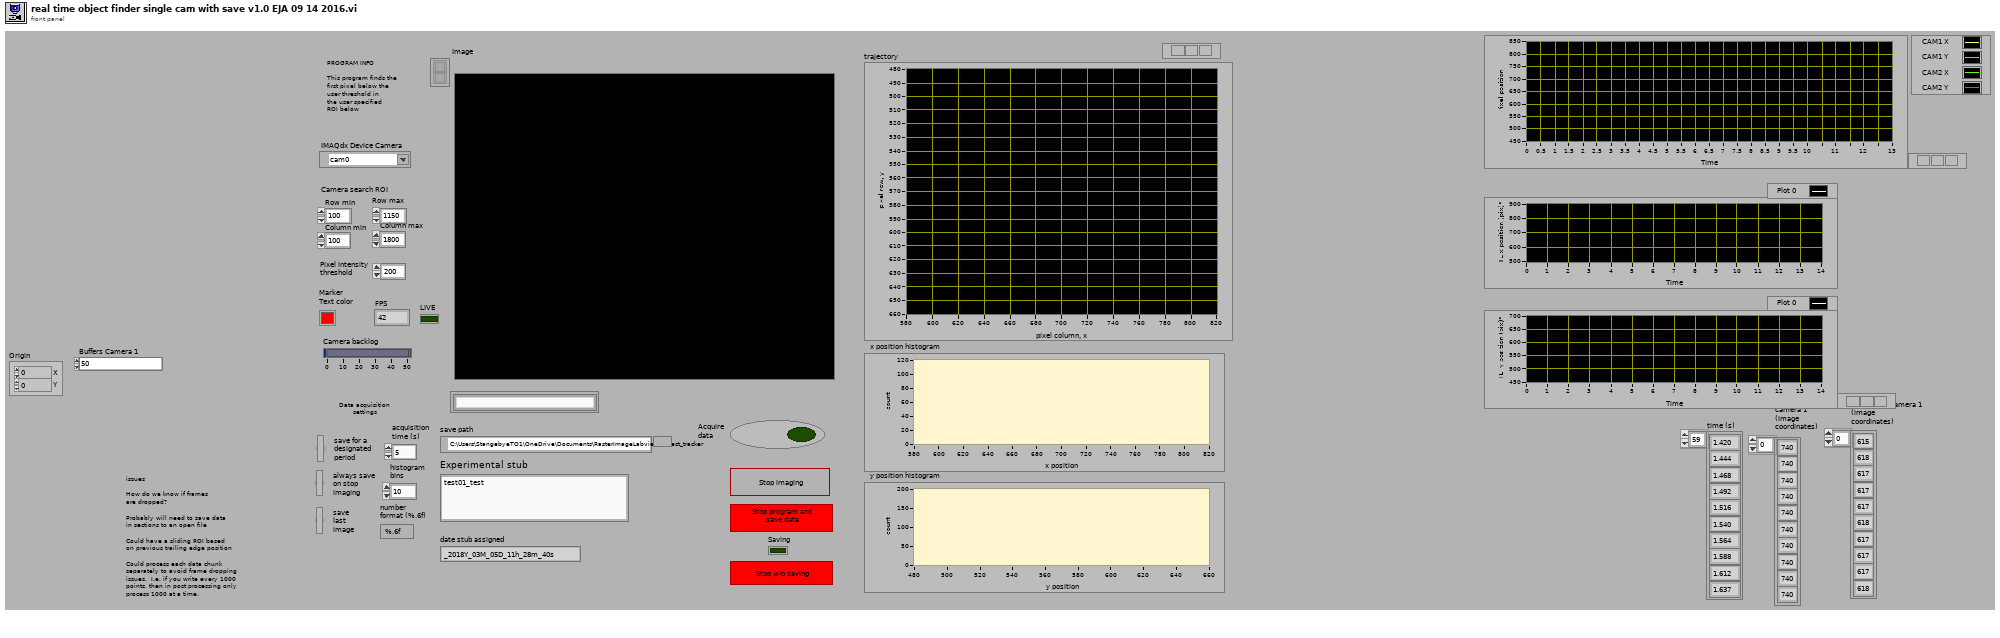
[diagram p1: front panel]
types:
  T1 = cluster{"X Values":dbl[], "Histogram: h(x)":i32[]}
  T2 = typedef "IMAQdx.ctl" = refnum<k21>
  T3 = typedef "IMAQ Image.ctl" = refnum<image>
  T4 = typedef "NI_Vision_Acquisition_Software.lvlib/IMAQdx Buffer Number Mode.ctl" = enum32{"Next", "Last", "Buffer Number", "Every", "Last New"}
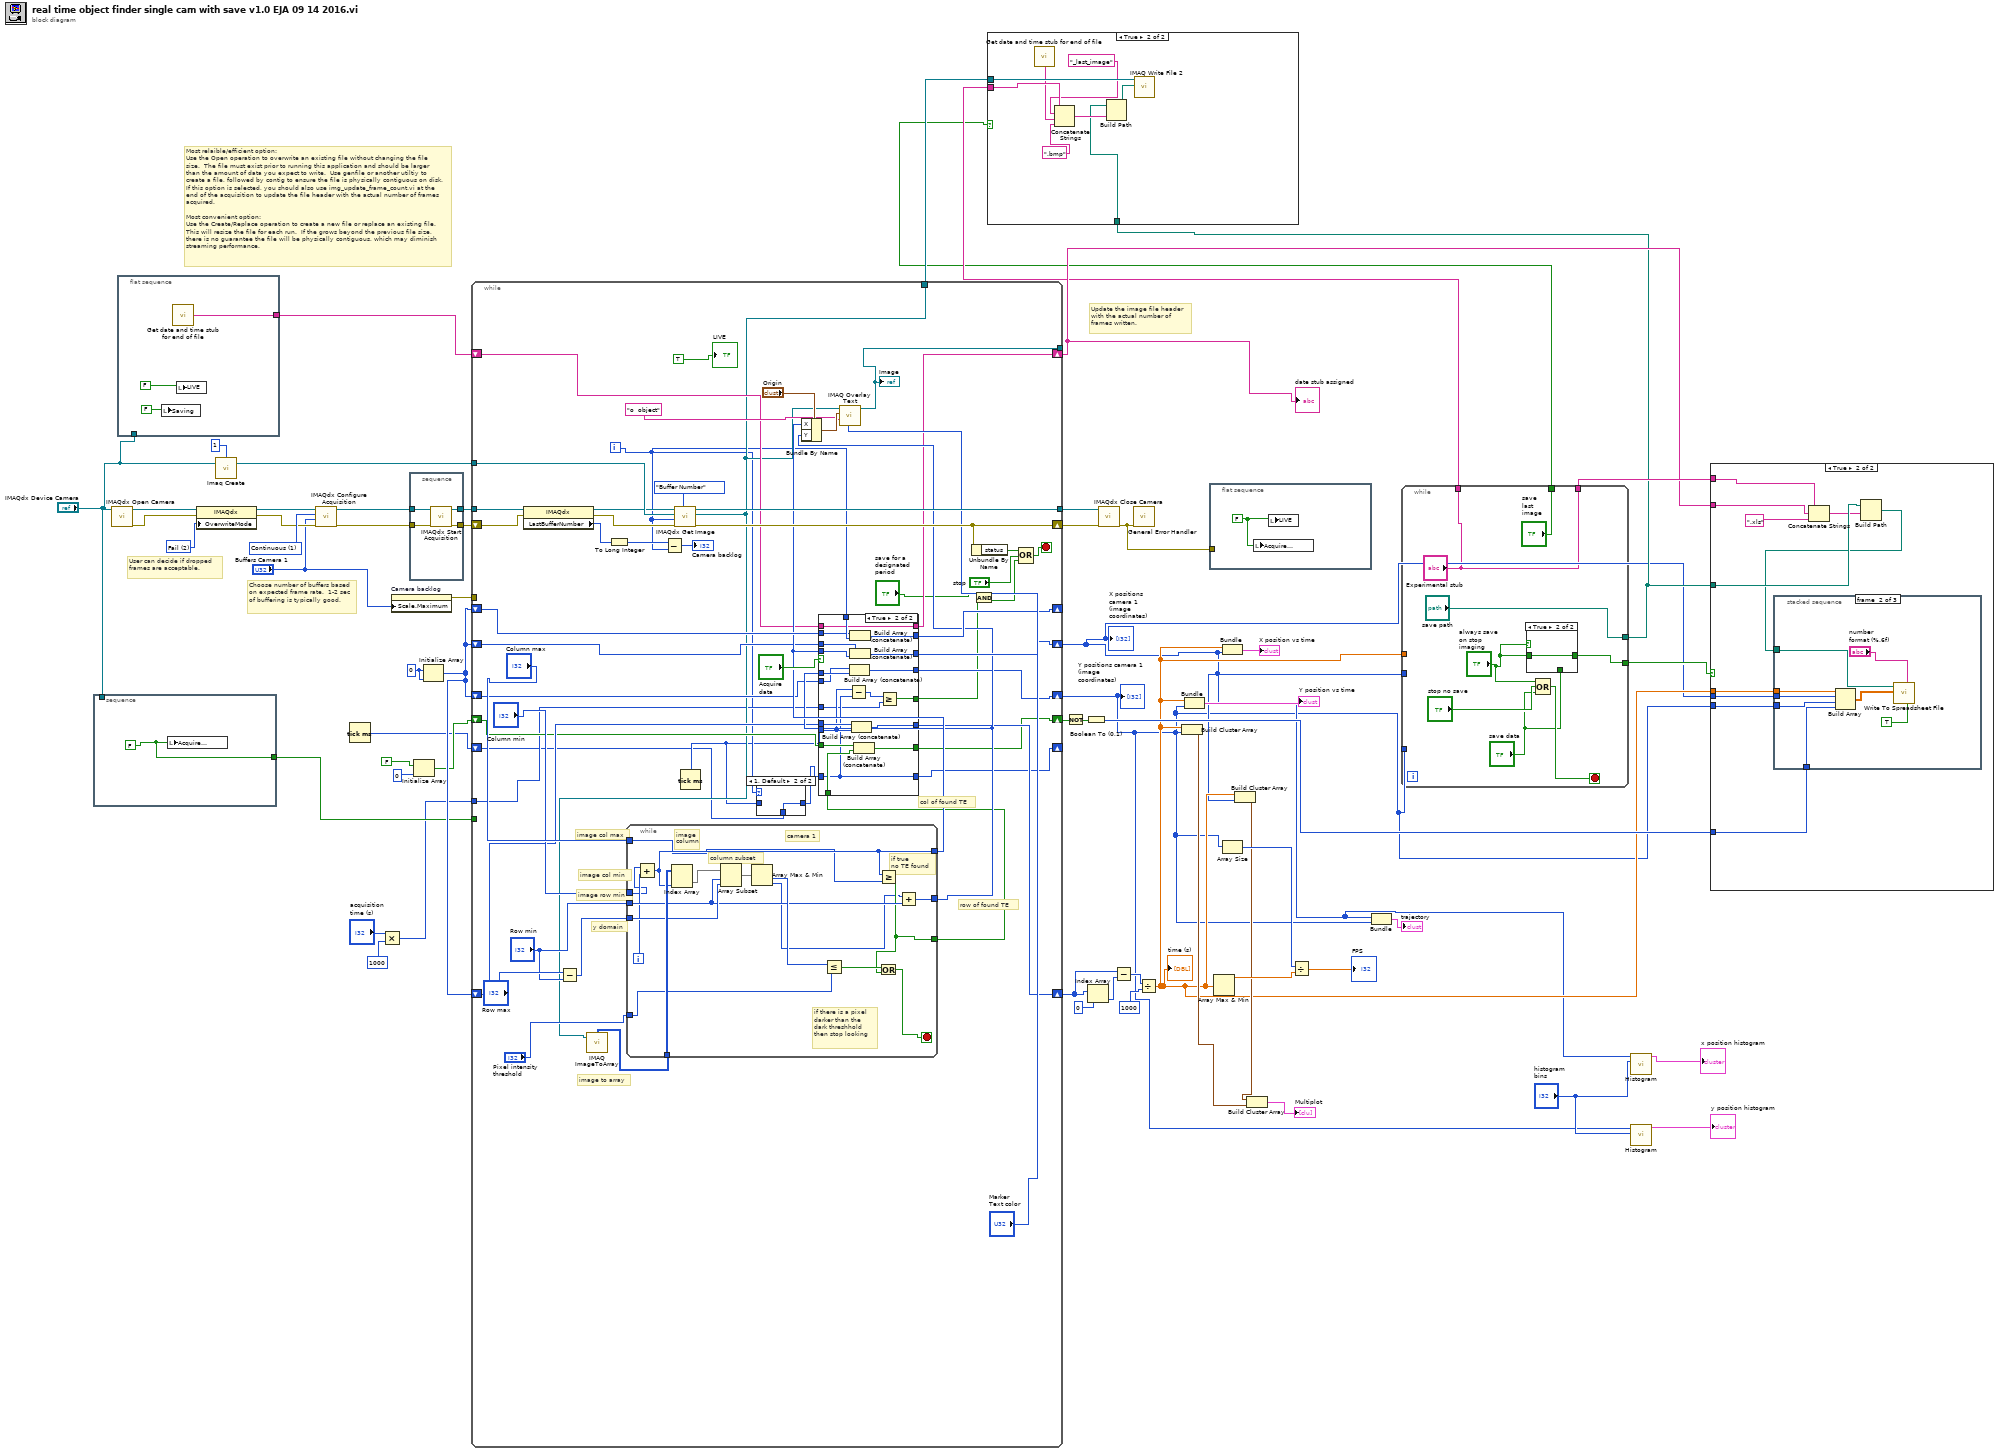
[diagram p0: block diagram]
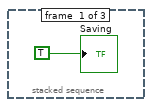
[diagram p4: hidden frame]
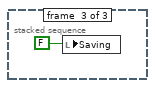
[diagram p5: hidden frame]
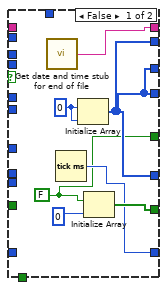
[diagram p8: hidden frame]
diagram:
  w28 = 0
  w52 = u32 2 items=["Get Oldest"=0, "Fail"=2, "Get Newest"=3] ("OverwriteMode")
  w58 = u32 1 items=["One Shot", "Continuous"] ("Continuous ?")
  # "Update the image file header with the actual number of frames written."
  # "Choose number of buffers based on expected frame rate.  1-2 sec of buffering is typically good."
  # "User can decide if dropped frames are acceptable."
  # "Most relaible/efficient option:\nUse the Open operation to overwrite an existing file without changing the file size.  The file must exist prior to running this application and should be larger than the amount of data you expect to write.  Use genfile or another utiltiy to create a file, followed by contig to ensure the file is physically contiguous on disk.  If this option is selected, you should also use img_update_frame_count.vi at the end of the acquisition to update the file header with the actual number of frames acquired. \n\nMost convenient option:\nUse the Create/Replace operation to create a new file or replace an existing file. This will resize the file for each run.  If the grows beyond the previous file size, there is no guarantee the file will be physically contiguous, which may diminish streaming performance."
  n1 = stacked-sequence {
    tunnel: "IMAQdx Device Camera" -> [_]
    tunnel: [w60] -> w12
    frame #0 {
      w60 = FALSE
      n2 = local write "Acquire\ndata"(w60) -> ()
    }
  }
  n3 = call <vilib>:"IMAQdx Open Camera.vi"("Session In"="IMAQdx Device Camera") -> ("error out"=w48:errorcluster, "Session Out"=w47:T2)  [unwired: 2 in, 7 out]
  n4 = flat-sequence {
    tunnel: "IMAQdx Device Camera" -> [_]
    tunnel: [w61] -> w27
    frame #0 {
      n5 = local write "Saving"(FALSE) -> ()
      n6 = call "Get date and time stub for end of file.vi"() -> ("date and time stub"=w61:string)
      n7 = local write "LIVE"(FALSE) -> ()
    }
  }
  n8 = property class="IMAQdx"(reference=w47, error in=w48, "OverwriteMode"=w52) -> (reference out=w50:T2, error out=w49:errorcluster)
  n9 = call "Imaq Create"("Border Size"=1, "Image Name"="IMAQdx Device Camera") -> ("New Image"=w59:T3)  [unwired: 2 in, 2 out]
  n10 = call <vilib>:"IMAQdx Configure Acquisition.vi"("error in"=w49, "Number of Buffers"="Buffers Camera 1", "Continuous?"=w58, "Session In"=w50) -> ("error out"=w44:errorcluster, "Session Out"=w51:T2)  [unwired: 6 out]
  n11 = Tick Count (ms)() -> (millisecond timer value=w6:u32)
  n12 = Multiply(x="acquisition \ntime (s)", y=1000) -> (x*y=w7:i32)
  n13 = property on="Camera backlog" class="Slide (strict)"("Scale.Maximum"="Buffers Camera 1") -> (error out=w46:errorcluster)  [unwired: 2 in, 1 out]
  n14 = stacked-sequence {
    tunnel: [w67] -> w57
    tunnel: [w66] -> w56
    tunnel: w51 -> [w65]
    tunnel: w44 -> [w64]
    frame #0 {
      n15 = call <vilib>:"IMAQdx Start Acquisition.vi"("error in"=w64, "Session In"=w65) -> ("error out"=w67:errorcluster, "Session Out"=w66:T2)  [unwired: 8 out]
    }
  }
  n16 = Initialize Array(FALSE, 0) -> (w19:bool[])
  n17 = Initialize Array(w28, w28) -> (w25:i32[])
  n18 = while {
    tunnel: [w115] -> w54
    tunnel: w56 -> [w118]
    tunnel: w59 -> [w116]
    tunnel: [w104] -> _
    shift-right: [w114] -> w53
    shift-left: w57 -> [w117]
    tunnel: w46 -> [_]
    shift-right: [w91] -> _
    shift-left: w25 -> [w92]
    shift-right: [w89] -> w5
    shift-left: w25 -> [w88]
    shift-right: [w86] -> w1
    shift-left: w25 -> [w85]
    shift-right: [w84] -> w38
    shift-left: w25 -> [w83]
    shift-right: [w81] -> w26
    shift-left: w27 -> [w82]
    shift-right: [w79] -> w24
    shift-left: w19 -> [w80]
    tunnel: [w77] -> w17
    tunnel: w12 -> [_]
    shift-right: [w76] -> _
    shift-left: w6 -> [w68]
    tunnel: w7 -> [w75]
    i -> [w71]
    stop <- w120 stop-if-true
    # "image col min"
    # "image col max"
    # "image row min"
    # "row of found TE"
    # "col of found TE"
    # "y domain"
    # "image to array"
    n19 = property class="IMAQdx"(reference=w118, error in=w117) -> (reference out=w111:T2, error out=w112:errorcluster, "LastBufferNumber"=w108:u32)
    n20 = Subtract(x="Row max", y="Row min") -> (x-y=w96:i32)
    n21 = To Long Integer(number=w108) -> (32bit integer=w107:i32)
    n22 = Subtract(x=w107, y=w71) -> (x-y=→"Camera backlog":i32)
    n23 = call <vilib>:"IMAQdx Get Image.vi"("Buffer Number Mode (Next)"=IMAQdx_Buffer_Number_Mode."Buffer Number", "error in"=w112, "Buffer Number In"=w71, "Image In"=w116, "Session In"=w111) -> ("error out"=w114:errorcluster, "Image Out"=w77:T3, "Session Out"=w115:T2)  [unwired: 1 in, 3 out]
    n24 = call "IMAQ ImageToArray"("Image"=w77) -> ("Image Pixels (U8)"=w105:u8[][])  [unwired: 2 in, 5 out]
    n25 = while {
      tunnel: "Row min" -> [w159]
      tunnel: [w158] -> w90
      tunnel: [w160] -> w87
      tunnel: w96 -> [w162]
      tunnel: w105 -> [w164]
      tunnel: "Column max" -> [w150]
      tunnel: "Column min" -> [w151]
      tunnel: [w155] -> w78
      tunnel: "Pixel intensity\nthreshold" -> [w153]
      i -> [w152]
      stop <- w156 stop-if-true
      # "if true\nno TE found"
      # "camera 1"
      # "if there is a pixel\ndarker than the\ndark threshhold\nthen stop looking"
      # "column subset"
      # "image\ncolumn"
      n26 = Add(x=w151, y=w152) -> (x+y=w158:i32)
      n27 = Index Array(array=w164, index (col)=w158) -> (element=w163:u8[])  [unwired: 1 in]
      n28 = Array Subset(array=w163, index=w159, length=w162) -> (w161:u8[])
      n29 = Array Max & Min(array=w161) -> (min value=w165:u8, min index (indices)=w154:i32)  [unwired: 2 out]
      n30 = Less Or Equal?(x=w165, y=w153) -> (x <= y?=w157:bool)
      n31 = Greater Or Equal?(x=w158, y=w150) -> (x >= y?=w155:bool)
      n32 = Or(x=w157, y=w155) -> (x .or. y?=w156:bool)
      n33 = Add(x=w154, y=w159) -> (x+y=w160:i32)
    }
    n34 = Tick Count (ms)() -> (millisecond timer value=w70:u32)
    n35 = case shown="1, Default" w71 {
      tunnel: w70 -> [w121 _]
      tunnel: [w121 w122] -> w69
      tunnel: w68 -> [_ w122]
      frame 0 {
      }
      frame 1, Default {
      }
    }
    n36 = Bundle By Name(cluster="Origin", "X"=w90, "Y"=w87) -> (w102:cluster{"X":i32, "Y":i32})
    n37 = case shown="True" "Acquire\ndata" {
      tunnel: w71 -> [_ w149]
      tunnel: w92 -> [_ w148]
      tunnel: [w127 w147] -> w91
      tunnel: w90 -> [_ w145]
      tunnel: [w127 w146] -> w89
      tunnel: w88 -> [_ w144]
      tunnel: w87 -> [_ w143]
      tunnel: [w127 w142] -> w86
      tunnel: w85 -> [_ w141]
      tunnel: w70 -> [_ w133]
      tunnel: [w127 w140] -> w84
      tunnel: w83 -> [_ w139]
      tunnel: [w128 w138] -> w81
      tunnel: w82 -> [_ w138]
      tunnel: w80 -> [_ w137]
      tunnel: w78 -> [_ w136]
      tunnel: [w125 w135] -> w79
      tunnel: w69 -> [_ w132]
      tunnel: [w124 w132] -> w76
      tunnel: w75 -> [_ w131]
      tunnel: [w123 w130] -> w74
      frame False {
        w123 = FALSE
        w129 = 0
        n38 = call "Get date and time stub for end of file.vi"() -> ("date and time stub"=w128:string)
        n39 = Tick Count (ms)() -> (millisecond timer value=w124:u32)
        n40 = Initialize Array(w129, w129) -> (w127:i32[])
        n41 = Initialize Array(w123, 0) -> (w125:bool[])
      }
      frame True {
        n42 = Subtract(x=w133, y=w132) -> (x-y=w134:u32)
        n43 = Build Array (concatenate)(w141, w143) -> (w142:i32[])
        n44 = Build Array (concatenate)(w148, w149) -> (w147:i32[])
        n45 = Build Array (concatenate)(w144, w145) -> (w146:i32[])
        n46 = Build Array (concatenate)(w139, w133) -> (w140:u32[])
        n47 = Build Array (concatenate)(w137, w136) -> (w135:bool[])
        n48 = Greater Or Equal?(x=w134, y=w131) -> (x >= y?=w130:bool)
      }
    }
    n49 = call "IMAQ Overlay Text"("Text Color (black)"="Marker\nText color", "String"="o  object", "Origin"=w102, "Image"=w77) -> ("Image Out"=w104:T3)  [unwired: 4 in, 3 out]
    "Image" <- w104
    n50 = Unbundle By Name(w114) -> ("status"=w119:bool)
    n51 = And(x="save for a \ndesignated \nperiod", y=w74) -> (x .and. y?=w73:bool)
    n52 = Compound Arithmetic op=OR(w119, "stop", w73) -> (w120:bool)
    "LIVE" <- TRUE
  }
  "X positions\ncamera 1\n(image \ncoordinates)" <- w5
  "Y positions camera 1 \n(image \ncoordinates)" <- w1
  "date stub assigned" <- w26
  n53 = Not(x=w24) -> (.not. x?=w21:bool[])
  n54 = Boolean To (0,1)(Boolean=w21) -> (0, 1=w20:i16[])
  n55 = Index Array(array=w38, index=0) -> (element=w39:u32)
  n56 = call <vilib>:"IMAQdx Close Camera.vi"("error in"=w53, "Session In"=w54) -> ("error out"=w43:errorcluster)  [unwired: 9 out]
  n57 = Subtract(x=w38, y=w39) -> (x-y=w33:u32[])
  n58 = call <vilib>:"General Error Handler.vi"("error in (no error)"=w43) -> ()  [unwired: 2 in, 13 out]
  n59 = Divide(x=w33, y=1000) -> (x/y=w11:dbl[])
  "time (s)" <- w11
  n60 = Build Cluster Array(w11, w1) -> (w30:cluster{dbl, i32}[])
  n61 = Bundle(w11, w1) -> (→"Y position vs time":cluster{dbl[], i32[]})  [unwired: 1 out]
  n62 = flat-sequence {
    tunnel: w43 -> [_]
    frame #0 {
      w166 = FALSE
      n63 = local write "Acquire\ndata"(w166) -> ()
      n64 = local write "LIVE"(w166) -> ()
    }
  }
  n65 = Array Max & Min(array=w11) -> (max value=w37:dbl)  [unwired: 3 out]
  n66 = Bundle(w11, w5) -> (→"X position vs time":cluster{dbl[], i32[]})  [unwired: 1 out]
  n67 = Array Size(array=w1) -> (size(s)=w36:i32)
  n68 = Build Cluster Array(w11, w5) -> (w31:cluster{dbl, i32}[])
  n69 = Build Cluster Array(w31, w30) -> (→"Multiplot":cluster{cluster{dbl, i32}[]}[])
  n70 = Divide(x=w36, y=w37) -> (x/y=→"FPS":dbl)
  n71 = Bundle(w5, w1) -> (→"trajectory":cluster{i32[], i32[]})  [unwired: 1 out]
  n72 = while {
    tunnel: w11 -> [_]
    tunnel: w5 -> [_]
    tunnel: w1 -> [_]
    tunnel: ["save path"] -> w15
    tunnel: ["Experimental stub"] -> w29
    tunnel: [w168] -> w18
    tunnel: ["Experimental stub"] -> w16
    tunnel: ["save\nlast\nimage"] -> w14
    stop <- w170 stop-if-true
    n73 = case shown="True" "always save\non stop\nimaging" {
      tunnel: [w175 w176] -> w168
      tunnel: "always save\non stop\nimaging" -> [_ w176]
      tunnel: "save data" -> [w175 _]
      frame False {
      }
      frame True {
      }
    }
    n74 = Compound Arithmetic op=OR("always save\non stop\nimaging", "stop no save", "save data") -> (w170:bool)
  }
  n75 = case shown="True" w14 {
    tunnel: w17 -> [_ w184]
    tunnel: w16 -> [_ w182]
    tunnel: w15 -> [_ w177]
    frame False {
    }
    frame True {
      n76 = call "Get date and time stub for end of file.vi"() -> ("date and time stub"=w180:string)
      n77 = Concatenate Strings(w182, "_last_image", w180, ".bmp") -> (w183:string)
      n78 = Build Path(base path=w177, name or relative path=w183) -> (appended path=w178:path)
      n79 = call-poly "IMAQ Write File 2"("File Path"=w178, "Image"=w184) -> ()  [unwired: 8 in, 2 out]
    }
  }
  n80 = call <vilib>:"Histogram.vi"("intervals"="histogram \nbins", "X"=w5) -> ("Histogram Graph"=→"x position histogram":T1)  [unwired: 6 in, 3 out]
  n81 = call <vilib>:"Histogram.vi"("intervals"="histogram \nbins", "X"=w1) -> ("Histogram Graph"=→"y position histogram":T1)  [unwired: 6 in, 3 out]
  n82 = case shown="True" w18 {
    tunnel: w11 -> [_ w194]
    tunnel: w5 -> [_ w193]
    tunnel: w1 -> [_ w192]
    tunnel: w29 -> [_ w190]
    tunnel: w15 -> [_ w189]
    tunnel: w26 -> [_ w186]
    tunnel: w20 -> [_ w185]
    frame False {
    }
    frame True {
      n83 = Concatenate Strings(w190, w186, ".xls") -> (w188:string)
      n84 = Build Path(base path=w189, name or relative path=w188) -> (appended path=w187:path)
      n85 = stacked-sequence {
        tunnel: w187 -> [_ w201 _]
        tunnel: w194 -> [_ w200 _]
        tunnel: w193 -> [_ w199 _]
        tunnel: w192 -> [_ w198 _]
        tunnel: w185 -> [_ w197 _]
        frame #0 {
          "Saving" <- TRUE
        }
        frame #1 {
          n86 = Build Array(w200, w199, w198, w197) -> (w196:dbl[][])
          n87 = call-poly <vilib>:"Write To Spreadsheet File.vi"("transpose? (no:F)"=TRUE, "format (%.3f)"="number\nformat (%.6f)", "2D data"=w196, "file path (dialog if empty)"=w201) -> ()  [unwired: 4 in, 1 out]
        }
        frame #2 {
          n88 = local write "Saving"(FALSE) -> ()
        }
      }
    }
  }
